vi "AM FGV All Step Data.vi"(7 "CMD":T1, 8 "error in (no error)":errorcluster, 10 "current Step":i32, 11 "Proc Data in":dbl[][](array[numeric])) -> (0 "error out":errorcluster, 3 "Proc Data Out":cluster{"SG COLD":dbl[][]})   [LabVIEW 2020]
uses:
  support/PCT FGV CMD.ctl
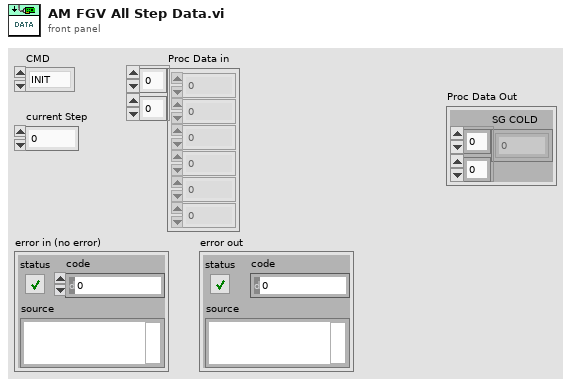
[diagram p1: front panel]
types:
  T1 = typedef "PCT FGV CMD.ctl" = enum16{"INIT", "GET", "SET"}
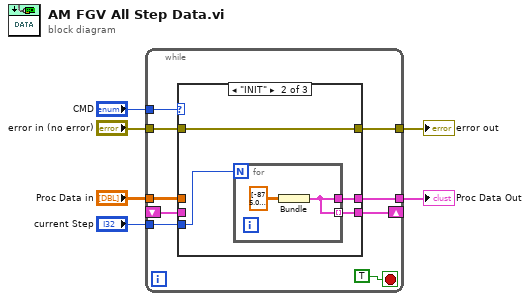
[diagram p0: block diagram]
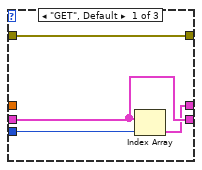
[diagram p2: hidden frame]
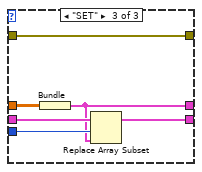
[diagram p3: hidden frame]
diagram:
  n1 = while {
    tunnel: "CMD" -> [w13]
    shift-right: [w12] -> _
    shift-left: _ -> [w11]
    tunnel: "error in (no error)" -> [w14]
    tunnel: [w15] -> w2
    tunnel: "current Step" -> [w9]
    tunnel: "Proc Data in" -> [w8]
    tunnel: [w7] -> w1
    stop <- TRUE stop-if-true
    n2 = case shown="\"INIT\"" w13 {
      tunnel: [w19 w23 w31] -> w15
      tunnel: [w18 w20 w30] -> w12
      tunnel: w14 -> [w19 w23 w31]
      tunnel: w11 -> [w18 _ w29]
      tunnel: w9 -> [w17 w21 w28]
      tunnel: w8 -> [_ _ w27]
      tunnel: [w16 w22 w26] -> w7
      frame "GET", Default {
        n3 = Index Array(array=w18, index=w17) -> (element=w16:cluster{"SG COLD":dbl[][]})
      }
      frame "INIT" {
        n4 = for {
          N: w21 -> [_]
          tunnel: [w24] -> w22
          tunnel: [w24] -> w20 mode=indexing
          n5 = Bundle("SG COLD"=dbl[][] [[-875.0, -601.0, -380.0, -223.0, -115.0, -47.0, -12.0, 0.0, -6.0, -20.0, -44.0, -68.0, -86.0, -99.0, -104.0, -94.0, -69.0, -28.0, 32.0, 110.0, 205.0, 325.0, 466.0, 640.0], [-906.0, -620.0, -391.0, -227.0, -117.0, -51.0, -15.0, 0.0, -2.0, -16.0, -38.0, -60.0, -77.0, -88.0, -91.0, -79.0, -53.0, -11.0, 50.0, 131.0, 227.0, 346.0, 490.0, 662.0], [-859.0, -595.0, -380.0, -223.0, -116.0, -49.0, -13.0, 0.0, -10.0, -31.0, -55.0, -81.0, -100.0, -115.0, -118.0, -110.0, -85.0, -46.0, 18.0, 97.0, 193.0, 311.0, 457.0, 631.0], [-832.0, -574.0, -364.0, -213.0, -108.0, -43.0, -10.0, 0.0, -9.0, -32.0, -56.0, -82.0, -101.0, -118.0, -121.0, -114.0, -91.0, -52.0, 9.0, 88.0, 183.0, 302.0, 447.0, 623.0], [-843.0, -583.0, -371.0, -217.0, -111.0, -47.0, -10.0, 0.0, -6.0, -27.0, -51.0, -77.0, -95.0, -111.0, -112.0, -106.0, -80.0, -41.0, 21.0, 99.0, 194.0, 312.0, 456.0, 632.0], [-867.0, -596.0, -378.0, -221.0, -114.0, -47.0, -12.0, 0.0, -7.0, -25.0, -48.0, -72.0, -90.0, -103.0, -106.0, -96.0, -70.0, -28.0, 34.0, 113.0, 206.0, 318.0, 462.0, 635.0]]) -> (w24:cluster{"SG COLD":dbl[][]})  [unwired: 1 in]
        }
      }
      frame "SET" {
        n6 = Bundle("Proc Data in"=w27) -> (w26:cluster{"Proc Data in":dbl[][]})  [unwired: 1 in]
        n7 = Replace Array Subset(array=w29, new element=w26, index=w28) -> (w30:cluster{"SG COLD":dbl[][]}[])
      }
    }
  }
  "Proc Data Out" <- w1
  "error out" <- w2
